vi "parse_PolynomialSegment_scalar.vi"(4 "error in":errorcluster, 7 "msg in":string) -> (0 "error out":errorcluster, 2 "Polynomial Segment":T1, 3 "msg out":string)   [LabVIEW 2018]
doc: "Parses a message into an acceleration"
uses:
  Google_Drive/Labview/Robot 3/Typedefs/Polynomial Segment typedef.ctl
  <userlib>/ROS for LabVIEW Software/ROS/MessageParsing/std_msgs/subs/parse_i32_scalar.vi
  <userlib>/ROS for LabVIEW Software/ROS/MessageParsing/std_msgs/subs/parse_float64_scalar.vi
  <userlib>/ROS for LabVIEW Software/ROS/MessageParsing/std_msgs/subs/parse_float64_array.vi
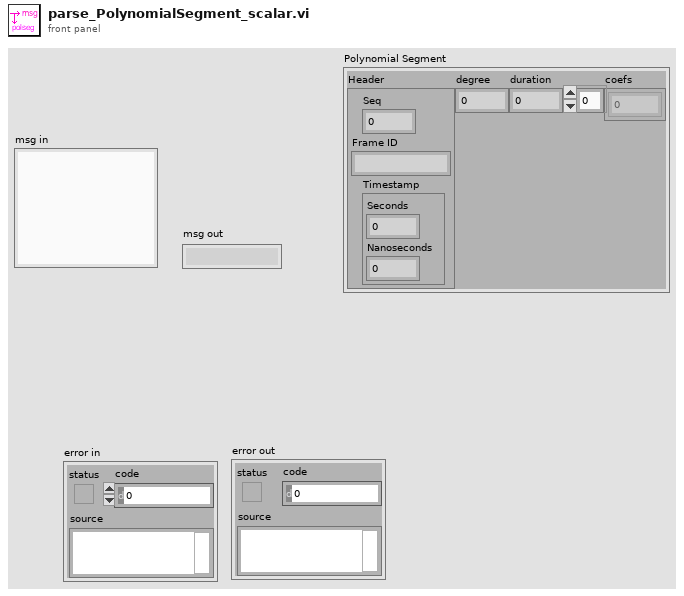
[diagram p1: front panel]
types:
  T1 = typedef "Polynomial Segment typedef.ctl" = cluster{"Header":cluster{"Seq":u32, "Frame ID":string, "Timestamp":cluster{"Seconds":i32, "Nanoseconds":i32}}, "degree":i32, "duration":dbl, "coefs":dbl[]}
  T2 = cluster{"Seq":u32, "Frame ID":string, "Timestamp":cluster{"Seconds":i32, "Nanoseconds":i32}}
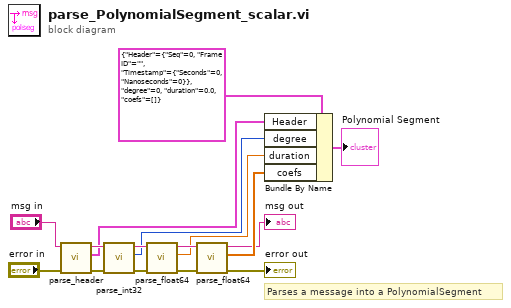
[diagram p0: block diagram]
diagram:
  # "Parses a message into a PolynomialSegment"
  n1 = call <userlib>:"parse_header.vi"("error in"="error in", "msg in"="msg in") -> ("error out"=w5:errorcluster, "Header"=w2:T2, "msg out"=w6:string)  [unwired: 3 in]
  n2 = call-poly <userlib>:"parse_int32.vi"("error in"=w5, "msg in"=w6) -> ("error out"=w10:errorcluster, "number"=w13:i32, "msg out"=w14:string)  [unwired: 3 in]
  n3 = call-poly <userlib>:"parse_float64.vi"("error in"=w10, "msg in"=w14) -> ("error out"=w9:errorcluster, "number"=w12:dbl, "msg out"=w15:string)  [unwired: 3 in]
  n4 = call-poly <userlib>:"parse_float64.vi"("error in"=w9, "msg in"=w15) -> ("error out"=→"error out":errorcluster, "number"=w11:dbl[], "msg out"=→"msg out":string)  [unwired: 3 in]
  n5 = Bundle By Name(cluster=T1 {"Header"={"Seq"=0, "Frame ID"="", "Timestamp"={"Seconds"=0, "Nanoseconds"=0}}, "degree"=0, "duration"=0.0, "coefs"=[]} ("PolynomialSegment"), "Header"=w2, "degree"=w13, "duration"=w12, "coefs"=w11) -> (→"Polynomial Segment":T1)
